vi "GetVIFromSubPanelName.vi"(0 "VI Reference in":refnum<vi>, 2 "delimiter (>>)":string=">>", 5 "Control Name":string, 11 "error in (no error)":errorcluster) -> (4 "VI Reference out":refnum<vi>, 6 "SubPanel VI Reference":refnum<vi>, 15 "error out":errorcluster)   [LabVIEW 2016]
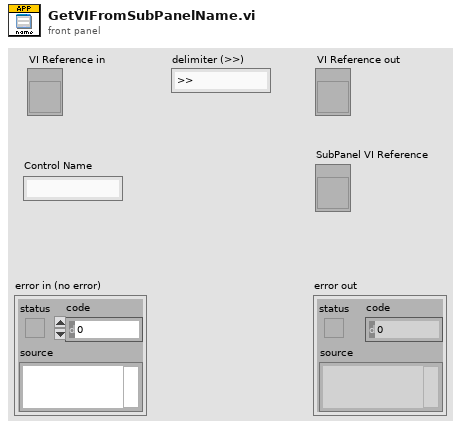
[diagram p1: front panel]
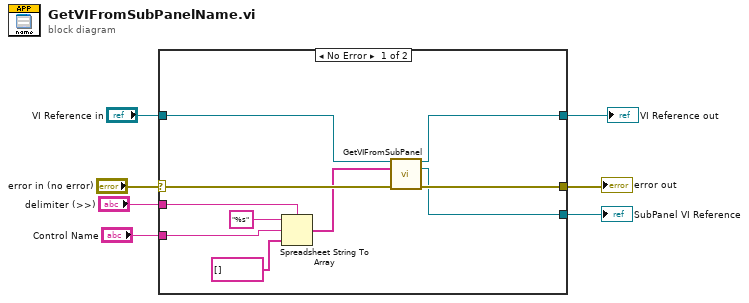
[diagram p0: block diagram]
diagram:
  n1 = case shown="No Error" "error in (no error)" {
    selector: "error in (no error)" -> [w15 w18]
    tunnel: "VI Reference in" -> [w17 w19]
    tunnel: [w16 w19] -> w5
    tunnel: [w14 w18] -> w4
    tunnel: "Control Name" -> [w11 _]
    tunnel: "delimiter (>>)" -> [w10 _]
    tunnel: [w8 _] -> w1
    frame No Error {
      n2 = Spreadsheet String To Array(delimiter (Tab)=w10, format string="%s", spreadsheet string=w11, array type (2D Dbl)=string[] []) -> (array=w9:string[])
      n3 = call "GetVIFromSubPanel.vi"("VI Reference in"=w17, "SubPanel Path"=w9, "error in (no error)"=w15) -> ("VI Reference out"=w16:refnum<vi>, "SubPanel VI Reference"=w8:refnum<vi>, "error out"=w14:errorcluster)  [unwired: 10 in]
    }
    frame Error {
    }
  }
  "error out" <- w4
  "SubPanel VI Reference" <- w1
  "VI Reference out" <- w5
